vi "convertForVelocity.vi"(9 "Wheel-val":dbl, 10 "encoder-val":dbl) -> (0 "Swerve Rotational Speed":dbl, 1 "Swerve Rel Angle":dbl, 2 "Wheel Speed":dbl, 3 "Wheel Distance":dbl, 4 "Swerve Rel Rotation":T1 {"SIN" format="%13.4f"; "COS" format="%13.4f"; "VALUE" format="%13.4f"}, 5 "Swerve Module State":T2={"Speed"=0.0, "Angle"={"VALUE"=0.0, "COS"=1.0, "SIN"=0.0}} {"Angle"."SIN" format="%13.4f"; "Angle"."COS" format="%13.4f"; "Angle"."VALUE" format="%13.4f"})   [LabVIEW 2020]
uses:
  <vilib>/Rock Robotics/WPI/ThirdParty/JAS_Junk/TrajLib/Trajectory_Library.lvlib
  <vilib>/Rock Robotics/WPI/ThirdParty/JAS_Junk/TrajLib/TypeDef/ROTATION2D.ctl
  <vilib>/Rock Robotics/WPI/ThirdParty/JAS_Junk/TrajLib/TypeDef/SWERVE_DRIVE_MODULE_STATE.ctl
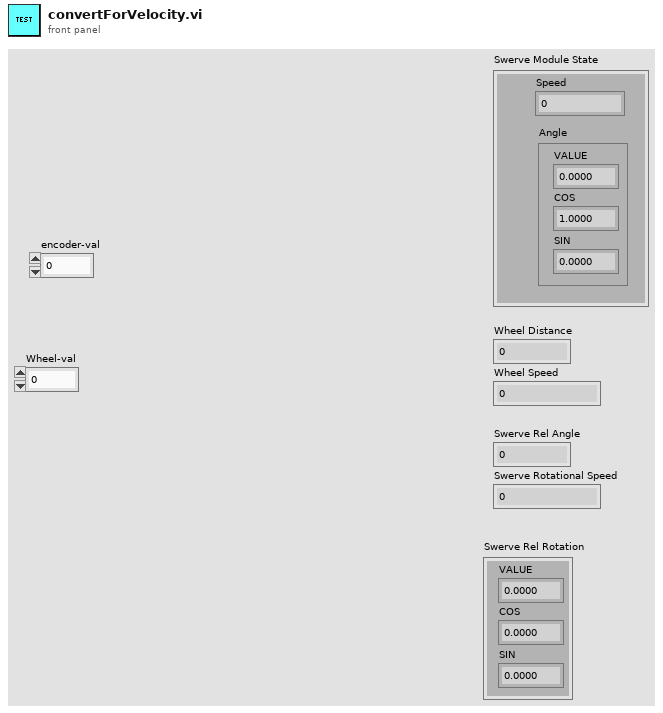
[diagram p1: front panel]
types:
  T1 = typedef "Trajectory_Library.lvlib/ROTATION2D.ctl" = cluster{"VALUE":dbl, "COS":dbl, "SIN":dbl}
  T2 = typedef "Trajectory_Library.lvlib/SWERVE_DRIVE_MODULE_STATE.ctl" = cluster{"Speed":dbl, "Angle":T1}
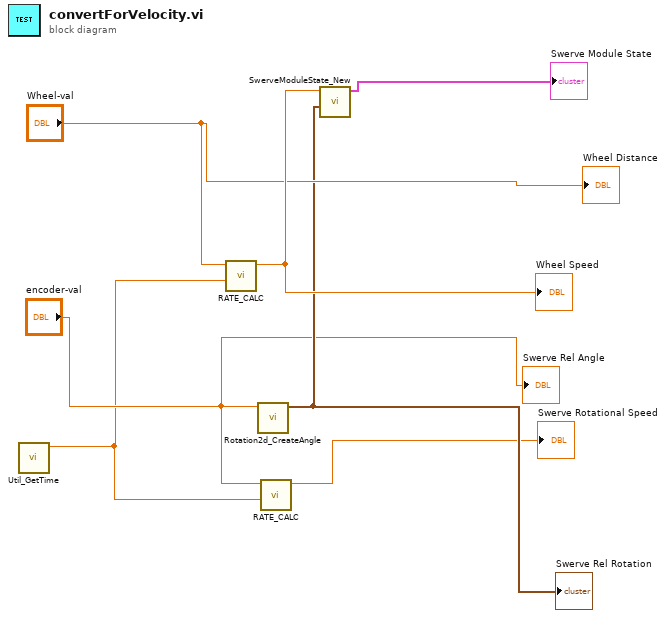
[diagram p0: block diagram]
diagram:
  n1 = call <vilib>:"Util_GetTime.vi"() -> ("FPGA_Time_Seconds"=w1:dbl)  [unwired: 9 in, 2 out]
  n2 = call "RATE_CALC.vi"("Time"=w1, "Input"="Wheel-val") -> ("Output"=w6:dbl)  [unwired: 9 in]
  "Wheel Speed" <- w6
  n3 = call <vilib>:"Rotation2d_CreateAngle.vi"("Angle"="encoder-val") -> ("ROTATION"=w4:T1)  [unwired: 10 in]
  "Swerve Rel Rotation" <- w4
  n4 = call "RATE_CALC.vi"("Time"=w1, "Input"="encoder-val") -> ("Output"=→"Swerve Rotational Speed":dbl)  [unwired: 9 in]
  n5 = call <vilib>:"SwerveModuleState_New.vi"("ROTATION"=w4, "Speed"=w6) -> ("SWERVE_DRIVE_MODULE_STATE"=→"Swerve Module State":T2)  [unwired: 9 in]
  "Wheel Distance" <- "Wheel-val"
  "Swerve Rel Angle" <- "encoder-val"
